vi "Average Detector for 1 s.vi"() -> ()   [LabVIEW 2016]
uses:
  <vilib>/DAQmx/read.llb/DAQmx Read (Analog 1D DBL 1Chan NSamp).vi
  <vilib>/Analysis/baseanly.llb/Mean (DBL).vi
  <vilib>/DAQmx/create/channels.llb/DAQmx Create Channel (AI-Voltage-Basic).vi
  <vilib>/DAQmx/configure/timing.llb/DAQmx Timing (Sample Clock).vi
  <vilib>/DAQmx/miscellaneous.llb/DAQmx Fill In Error Info.vi
  <vilib>/Analysis/NI_AALBase.lvlib
panel:
  out "mean":dbl format="%0.3f"
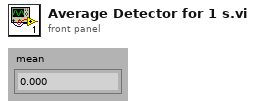
[diagram p1: front panel]
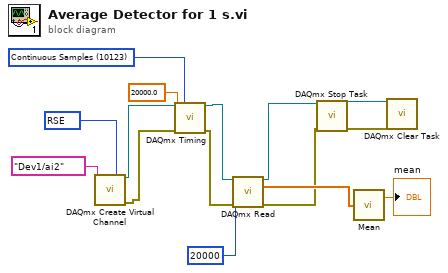
[diagram p0: block diagram]
diagram:
  w5 = 10123 items=["Finite Samples"=10178, "Continuous Samples"=10123, "Hardware Timed Single Point"=12522] ("sample mode")
  w12 = 10083 items=["default"=-1, "RSE"=10083, "NRSE"=10078, "Differential"=10106, "Pseudodifferential"=12529] ("input terminal configuration")
  n1 = call-poly <vilib>:"DAQmx Create Virtual Channel.vi"("input terminal configuration"=w12, "physical channels"=tag "Dev1/ai2") -> ("task out"=w7:refnum<k21>, "error out"=w10:errorcluster)  [unwired: 12 in]
  n2 = call-poly <vilib>:"DAQmx Timing.vi"("task/channels in"=w7, "sample mode"=w5, "rate"=20000.0, "error in"=w10) -> ("task out"=w8:refnum<k21>, "error out"=w9:errorcluster)  [unwired: 10 in]
  n3 = call-poly <vilib>:"DAQmx Read.vi"("task/channels in"=w8, "number of samples per channel"=20000, "error in"=w9) -> ("task out"=w3:refnum<k21>, "data"=w15:dbl[], "error out"=w4:errorcluster)  [unwired: 10 in]
  n4 = call <vilib>:"DAQmx Stop Task.vi"("task/channels in"=w3, "error in"=w4) -> ("task out"=w1:refnum<k21>, "error out"=w2:errorcluster)  [unwired: 12 in]
  n5 = call-poly <vilib>:"Mean.vi"("X"=w15) -> ("mean"=→"mean":dbl)  [unwired: 1 out]
  n6 = call <vilib>:"DAQmx Clear Task.vi"("task in"=w1, "error in"=w2) -> ()  [unwired: 13 in, 1 out]
